vi "Display array on Figure.vi"(1 "Y resolution":u32=1024, 2 "X resolution":u32=1024, 5 "format string":string, 6 "Image fit to":u8(ring) items=["Width", "Height"], 7 "Primary grid @ green":bool, 8 "Input array":dbl[][](array[numeric]), 9 "Primary Y":u8=1, 10 "Primary X":u8=1, 11 "Image reference":refnum<vi>) -> ()   [LabVIEW 2018]
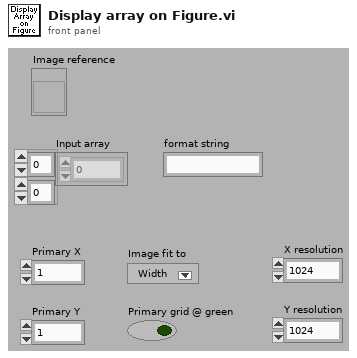
[diagram p1: front panel]
types:
  T1 = cluster{"horizontal":enum16{"left", "center", "right"}, "vertical":enum16{"top", "center", "bottom"}}
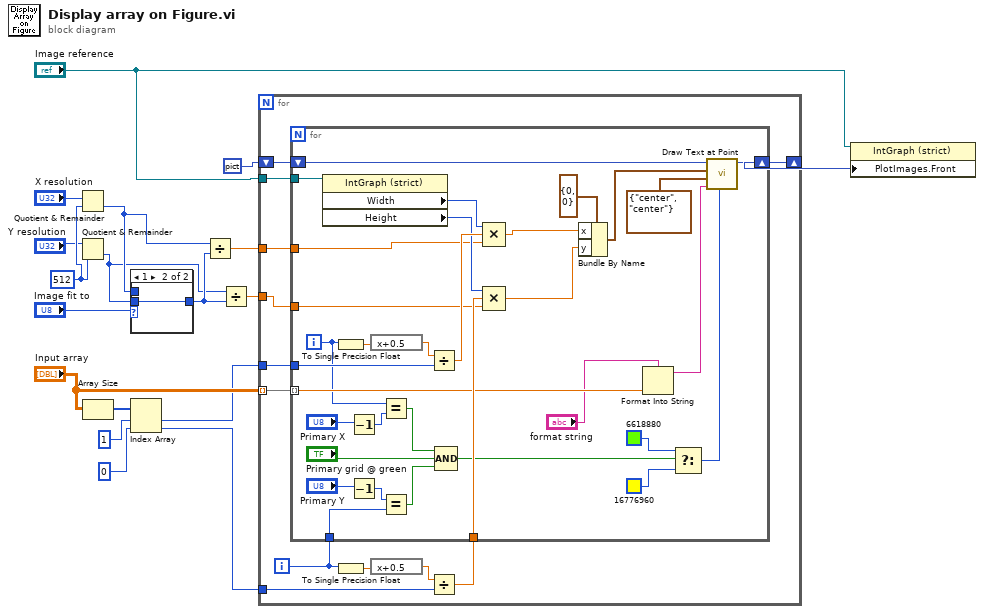
[diagram p0: block diagram]
diagram:
  w3 = u32 512 ("y")
  n1 = Quotient & Remainder(x="X resolution", y=w3) -> (floor(x/y)=w5:u32)  [unwired: 1 out]
  n2 = Quotient & Remainder(x="Y resolution", y=w3) -> (floor(x/y)=w1:u32)  [unwired: 1 out]
  n3 = Array Size(array="Input array") -> (size(s)=w15:i32[])
  n4 = case shown="1" "Image fit to" {
    tunnel: w5 -> [w19 _]
    tunnel: w1 -> [_ w20]
    tunnel: [w19 w20] -> w9
    frame 0, Default {
    }
    frame 1 {
    }
  }
  n5 = Index Array(array=w15, index #1=1 ("index"), index #2=0 ("index")) -> (element #1=w14:i32, element #2=w13:i32)
  n6 = Divide(x=w5, y=w9) -> (x/y=w6:dbl)
  n7 = Divide(x=w1, y=w9) -> (x/y=w7:dbl)
  n8 = for {
    shift-right: [w32] -> w18
    shift-left: picture data[5B] ("picture") -> [w31]
    tunnel: "Image reference" -> [w28]
    tunnel: "Input array" -> [w27] mode=indexing
    tunnel: w14 -> [w26]
    tunnel: w13 -> [w25]
    tunnel: w6 -> [w22]
    tunnel: w7 -> [w21]
    i -> [w24]
    n9 = To Single Precision Float(number=w24) -> (single precision float=w30:sgl)
    n10 = expression code="x+0.5"(w30) -> (w23:sgl)
    n11 = Divide(x=w23, y=w25) -> (x/y=w29:sgl)
    n12 = for {
      shift-right: [w59] -> w32
      shift-left: w31 -> [w58]
      tunnel: w29 -> [w57]
      tunnel: w28 -> [w54]
      tunnel: w27 -> [w53] mode=indexing
      tunnel: w26 -> [w52]
      tunnel: w24 -> [w47]
      tunnel: w22 -> [w34]
      tunnel: w21 -> [w33]
      i -> [w46]
      n13 = property on="Property Node" class="IntGraph (strict)"(reference=w54) -> ("Width"=w56:u32, "Height"=w55:u32)  [unwired: 1 in, 2 out]
      n14 = To Single Precision Float(number=w46) -> (single precision float=w62:sgl)
      n15 = Decrement(x="Primary X") -> (x-1=w38:u8)
      n16 = Decrement(x="Primary Y") -> (x-1=w37:u8)
      n17 = expression code="x+0.5"(w62) -> (w63:sgl)
      n18 = Equal?(x=w46, y=w38) -> (x = y?=w42:bool)
      n19 = Equal?(x=w37, y=w47) -> (x = y?=w44:bool)
      n20 = Divide(x=w63, y=w52) -> (x/y=w64:sgl)
      n21 = Compound Arithmetic op=AND(w42, "Primary grid @ green", w44) -> (w43:bool)
      n22 = Compound Arithmetic op=MULTIPLY(w56, w64, w34) -> (w36:dbl)
      n23 = Compound Arithmetic op=MULTIPLY(w55, w57, w33) -> (w35:dbl)
      n24 = Bundle By Name(cluster=cluster{"x":i16, "y":i16} {"x"=0, "y"=0} ("origin"), "x"=w36, "y"=w35) -> (w61:cluster{"x":i16, "y":i16})
      n25 = Format Into String(format string="format string", w53) -> (resulting string=w65:string)  [unwired: 2 in, 1 out]
      n26 = Select(t=u32 6618880 ("text color(black)"), s=w43, f=u32 16776960 ("text color(black)")) -> (s? t:f=w49:u32)
      n27 = call <vilib>:"Draw Text at Point.vi"("text color(black)"=w49, "text"=w65, "alignment(left, top)"=T1 {"horizontal"=enum."center", "vertical"=enum."center"}, "origin"=w61, "picture"=w58) -> ("new picture"=w59:picture)  [unwired: 5 in, 1 out]
    }
  }
  n28 = property on="Property Node" class="IntGraph (strict)"(reference="Image reference", "PlotImages.Front"=w18) -> ()  [unwired: 1 in, 2 out]
